vi "AlignTrigger.vi"(0 "log path in":path, 1 "triggerTimestamp":sgl format="%#_13g", 11 "error in (no error)":errorcluster, 12 "AcqRate":dbl) -> (4 "log path out":path, 15 "error out":errorcluster)   [LabVIEW 2015, in "BufferLogging.lvlib"]
uses:
  BufferLogging.lvlib
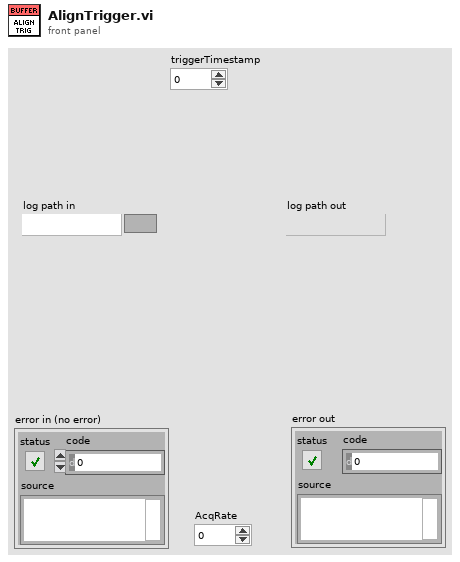
[diagram p1: front panel]
types:
  T1 = enum16{"open", "open or create", "create or replace", "create", "open (read-only)"}
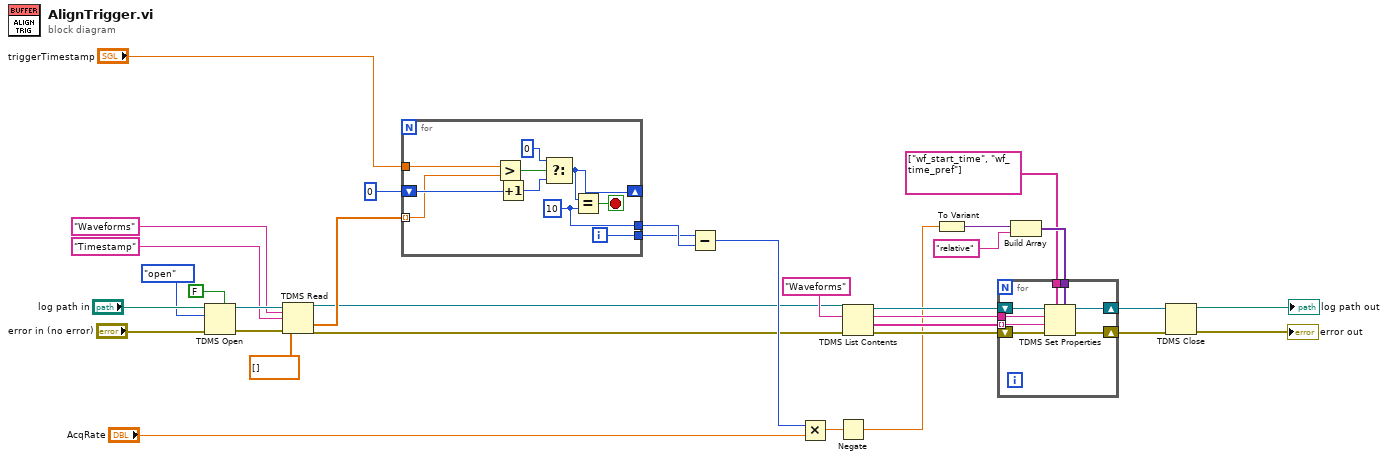
[diagram p0: block diagram]
diagram:
  n1 = TDMS Open(5:FALSE ("create index file? (T)"), 8:"error in (no error)", 10:T1."open" ("operation (0:open)"), 11:"log path in") -> (0:w16:errorcluster, 3:w17:refnum<k34>)  [unwired: 3 in]
  n2 = TDMS Read(0:w17, 5:"Waveforms" ("group name in"), 7:"Timestamp" ("group name in"), 11:w16, 12:sgl[] []) -> (4:w11:refnum<k34>, 10:w12:sgl[], 15:w10:errorcluster)  [unwired: 3 in, 3 out]
  n3 = for {
    tunnel: w12 -> [w37] mode=indexing
    tunnel: "triggerTimestamp" -> [w43]
    shift-right: [w40] -> _
    shift-left: 0 -> [w41]
    tunnel: [w38] -> w32
    tunnel: [w34] -> w5
    i -> [w34]
    stop <- w39 stop-if-true
    w38 = 10 ("y")
    n4 = Greater?(x=w43, y=w37) -> (0:w42:bool)
    n5 = Increment(x=w41) -> (x+1=w36:i32)
    n6 = Select(t=0 ("f"), s=w42, f=w36) -> (s? t:f=w40:i32)
    n7 = Equal?(x=w40, y=w38) -> (x = y?=w39:bool)
  }
  n8 = Subtract(x=w5, y=w32) -> (x-y=w31:i32)
  n9 = Multiply(x=w31, y="AcqRate") -> (x*y=w25:dbl)
  n10 = Negate(x=w25) -> (-x=w3:dbl)
  n11 = TDMS List Contents(4:w10, 6:"Waveforms" ("group name in"), 7:w11) -> (0:w26:errorcluster, 1:w22:string[], 2:w23:string, 3:w27:refnum<k34>)
  n12 = To Variant(anything=w3) -> (Variant=w2:variant)
  n13 = Build Array(w2, "relative") -> (w28:variant[])
  n14 = for {
    tunnel: string[] ["wf_start_time", "wf_time_pref"] -> [w47]
    tunnel: w28 -> [w48]
    shift-right: [w49] -> w9
    shift-left: w26 -> [w51]
    tunnel: w23 -> [w46]
    tunnel: w22 -> [w45] mode=indexing
    shift-right: [w44] -> w7
    shift-left: w27 -> [w50]
    n15 = TDMS Set Properties(5:w48, 7:w47, 8:w51, 9:w45, 10:w46, 11:w50) -> (0:w49:errorcluster, 3:w44:refnum<k34>)  [unwired: 2 out]
  }
  n16 = TDMS Close(8:w9, 11:w7) -> (0:→"error out":errorcluster, 3:→"log path out":path)
